vi "Log Errors.vi"(1 "Error Queue":refnum<queue>, 2 "Error Notifier":refnum<notifier>, 3 "Log File Cluster":T1) -> ()   [LabVIEW 2016]
uses:
  Log File Cluster.ctl
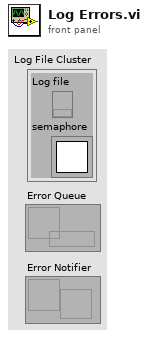
[diagram p1: front panel]
types:
  T1 = typedef "Log File Cluster.ctl" = cluster{"Log file":refnum<k34>, "semaphore":T2}
  T2 = typedef "Semaphore RefNum" = refnum<k1>
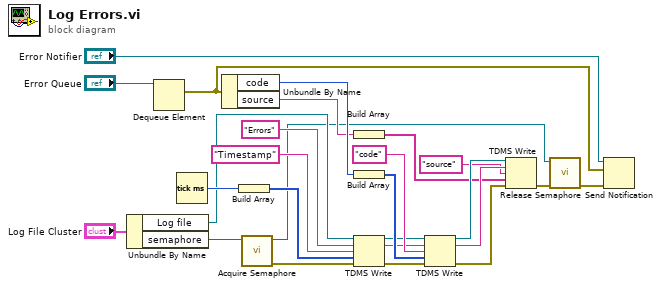
[diagram p0: block diagram]
diagram:
  n1 = Unbundle By Name("Log File Cluster") -> ("Log file"=w8:refnum<k34>, "semaphore"=w7:T2)
  n2 = Dequeue Element(queue="Error Queue") -> (element=w1:errorcluster)  [unwired: 2 in, 3 out]
  n3 = Tick Count (ms)() -> (millisecond timer value=w16:u32)
  n4 = Unbundle By Name(w1) -> ("code"=w26:i32, "source"=w21:string)
  n5 = Build Array(w16) -> (w15:u32[])
  n6 = call <vilib>:"Acquire Semaphore.vi"("semaphore"=w7) -> ("error out"=w6:errorcluster, "semaphore out"=w4:T2)  [unwired: 4 in, 1 out]
  n7 = Build Array(w21) -> (w20:string[])
  n8 = Build Array(w26) -> (w25:i32[])
  n9 = TDMS Write(0:w8, 5:"Errors" ("group name in (Untitled)"), 7:"Timestamp", 9:w15, 11:w6) -> (4:w10:refnum<k34>, 6:w12:string, 15:w11:errorcluster)  [unwired: 1 in, 1 out]
  n10 = TDMS Write(0:w10, 5:w12, 7:"code", 9:w25, 11:w11) -> (4:w24:refnum<k34>, 6:w23:string, 15:w22:errorcluster)  [unwired: 1 in, 1 out]
  n11 = TDMS Write(0:w24, 5:w23, 7:"source", 9:w20, 11:w22) -> (15:w5:errorcluster)  [unwired: 1 in, 3 out]
  n12 = call <vilib>:"Release Semaphore.vi"("error in (no error)"=w5, "semaphore"=w4) -> ("error out"=w2:errorcluster)  [unwired: 4 in, 1 out]
  n13 = Send Notification(notification=w1, notifier="Error Notifier", error in (no error)=w2) -> ()  [unwired: 2 out]
